vi "列表索引数组去重.vi"(1 "待去重数组":i32[](array[numeric])) -> (0 "数组输出":i32[](array[numeric]))   [LabVIEW 2015]
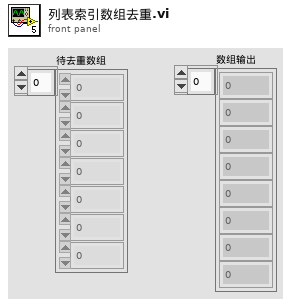
[diagram p1: front panel]
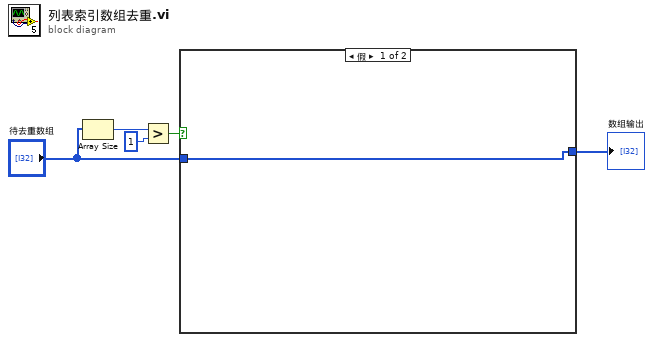
[diagram p0: block diagram]
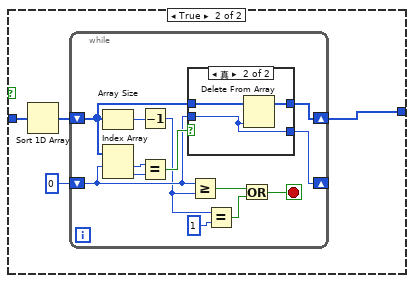
[diagram p2: hidden frame]
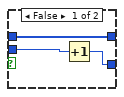
[diagram p3: hidden frame]
diagram:
  n1 = Array Size(array="待去重数组") -> (size(s)=w2:i32)
  n2 = Greater?(x=w2, y=1 ("大小")) -> (0:w5:bool)
  n3 = case shown="假" w5 {
    tunnel: "待去重数组" -> [w6 w9]
    tunnel: [w6 w7] -> w1
    frame False {
    }
    frame True {
      n4 = Sort 1D Array(array=w9) -> (sorted array=w8:i32[])
      n5 = while {
        shift-right: [w21] -> _
        shift-left: 0 -> [w18]
        shift-right: [w19] -> w7
        shift-left: w8 -> [w17]
        stop <- w15 stop-if-true
        n6 = Array Size(array=w17) -> (size(s)=w16:i32)
        n7 = Index Array(array=w17, index #1=w18) -> (element #1=w20:i32, element #2=w22:i32)  [unwired: 1 in]
        n8 = Decrement(x=w16) -> (x-1=w12:i32)
        n9 = Equal?(x=w20, y=w22) -> (x = y?=w23:bool)
        n10 = case shown="真" w23 {
          tunnel: [w25 w27] -> w21
          tunnel: w18 -> [w26 w27]
          tunnel: w17 -> [w24 w29]
          tunnel: [w24 w28] -> w19
          frame False {
            n11 = Increment(x=w26) -> (x+1=w25:i32)
          }
          frame True {
            n12 = Delete From Array(array=w29, index=w27) -> (array with subset deleted=w28:i32[])  [unwired: 1 in, 1 out]
          }
        }
        n13 = Greater Or Equal?(x=w18, y=w12) -> (x >= y?=w14:bool)
        n14 = Equal?(x=w12, y=1) -> (x = y?=w13:bool)
        n15 = Or(x=w14, y=w13) -> (x .or. y?=w15:bool)
      }
    }
  }
  "数组输出" <- w1
